vi "Get VI Error Out Value.vi"(8 "error in":errorcluster, 11 "vi reference in":refnum<vi>) -> (0 "error out":errorcluster, 2 "vi error out":errorcluster, 3 "dup vi reference":refnum<vi>)   [LabVIEW 2011, in "VITesterUtilities.lvlib"]
uses:
  Libraries/VITesterUtilities.lvlib
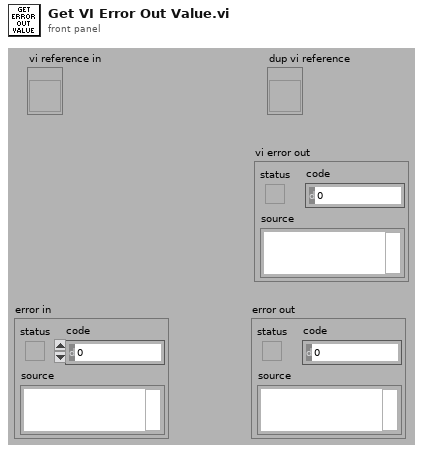
[diagram p1: front panel]
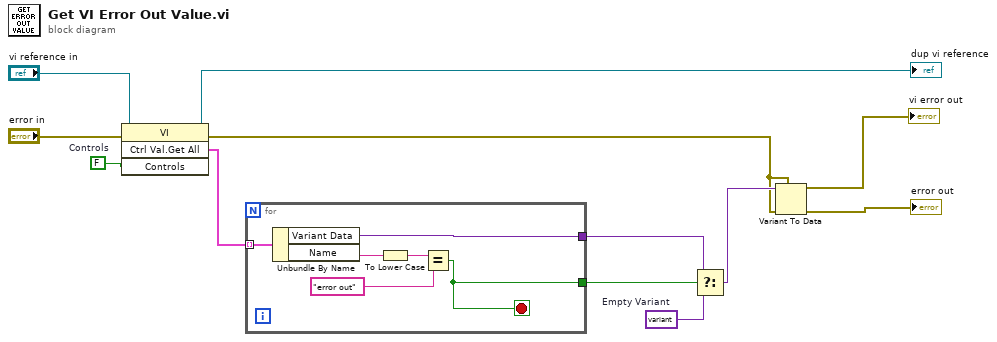
[diagram p0: block diagram]
diagram:
  w7 = variant  # Empty Variant
  w11 = FALSE  # Controls
  n1 = invoke class="VI" method="Ctrl Val.Get All"(reference="vi reference in", error in="error in", "Controls"=w11) -> (reference out=→"dup vi reference":refnum<vi>, error out=w3:errorcluster, "Get All Control Values Variant"=w10:cluster{"Name":string, "Variant Data":variant}[])  [unwired: 1 in, 1 out]
  n2 = for {
    tunnel: w10 -> [w18] mode=indexing
    tunnel: [w14] -> w8
    tunnel: [w13] -> w9
    stop <- w13 stop-if-true
    n3 = Unbundle By Name(w18) -> ("Variant Data"=w14:variant, "Name"=w17:string)
    n4 = To Lower Case(string=w17) -> (all lower case string=w15:string)
    n5 = Equal?(x=w15, y="error out" ("Control Name")) -> (x = y?=w13:bool)
  }
  n6 = Select(t=w8, s=w9, f=w7) -> (s? t:f=w4:variant)
  n7 = Variant To Data(error in=w3, type=w3, Variant=w4) -> (data=→"vi error out":errorcluster, error out=→"error out":errorcluster)
